vi "PROJE (1).vi"() -> ()   [LabVIEW 2017]
panel:
  in  "Kaydet":bool
  in  "Çıkış":bool
  in  "Path":path
  out "Waveform Chart":dbl(graph)
  in  "SENSOR NEVEL":dbl(slide) scale=0.0..100.0
  out "Tank":dbl(slide) scale=0.0..100.0
  out "tank  hızı":dbl
  in  "tekrar sayısı":dbl
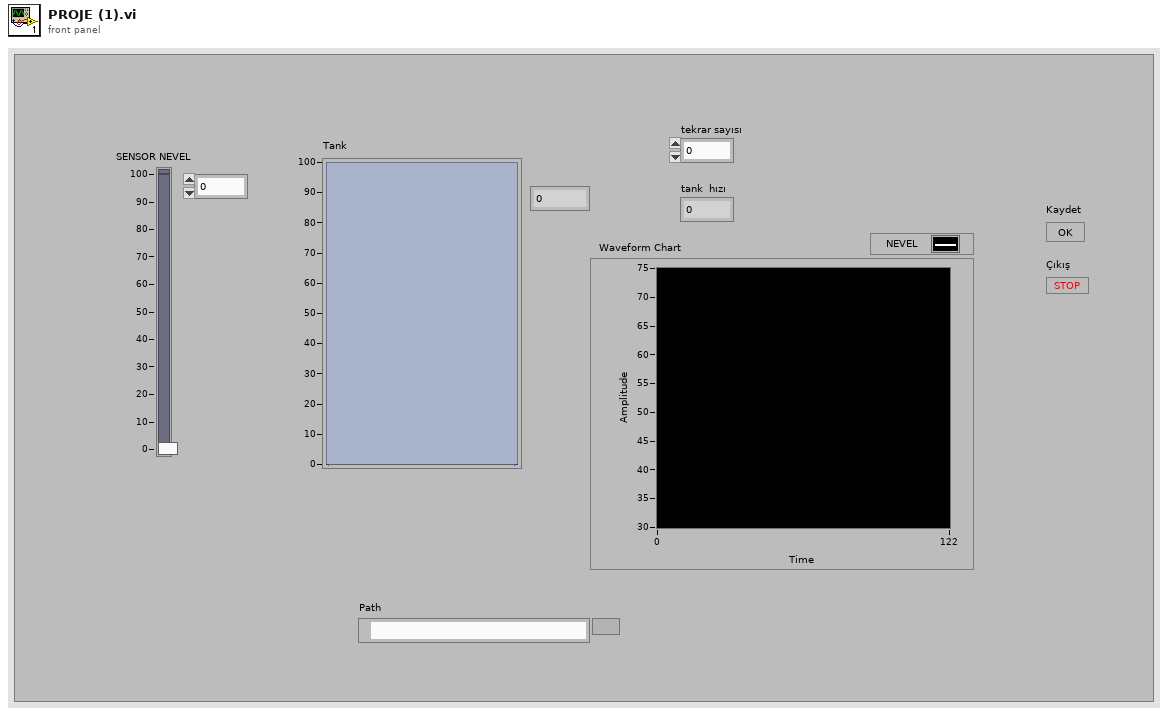
[diagram p1: front panel]
types:
  T1 = enum16{"open", "replace", "create", "open or create", "replace or create", "replace or create with confirmation"}
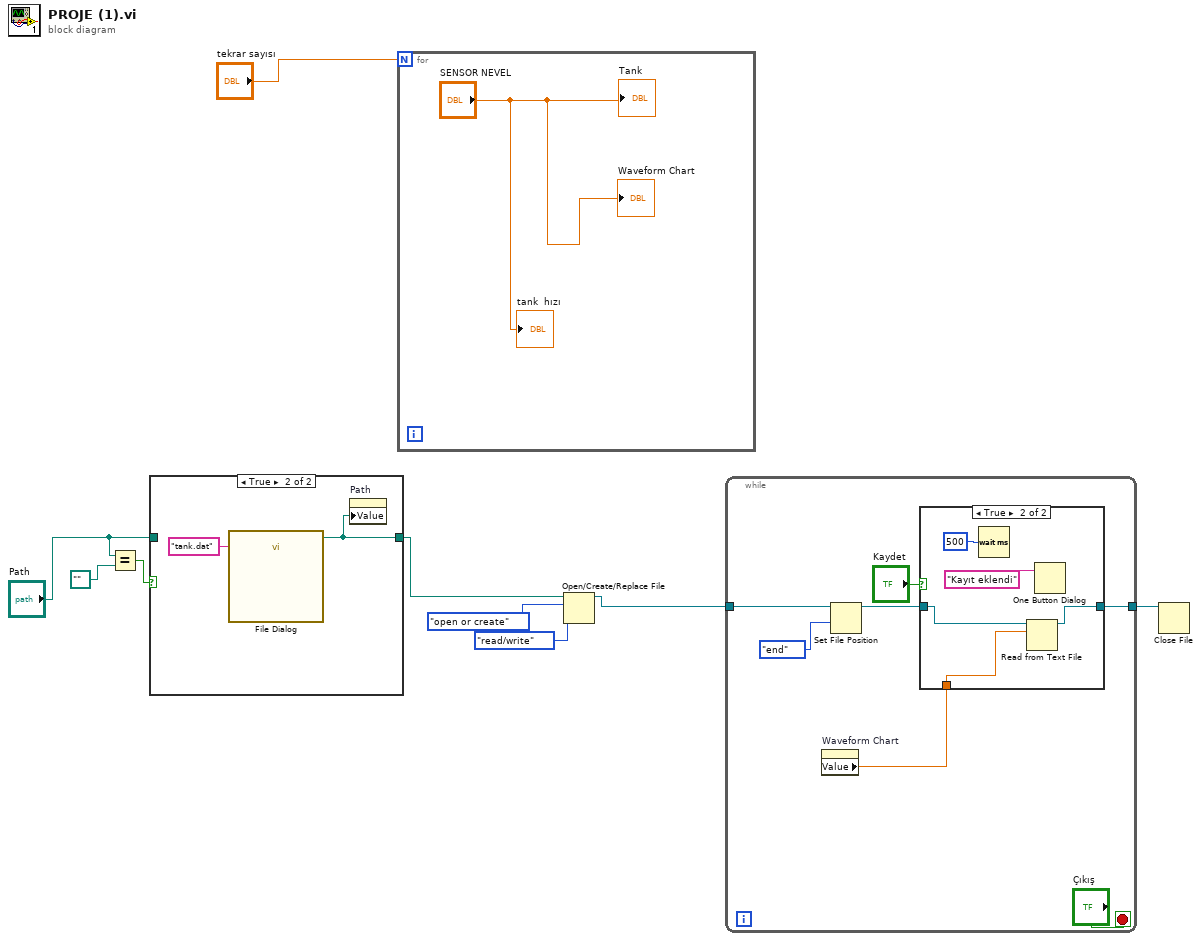
[diagram p0: block diagram]
diagram:
  n1 = Equal?(x="Path", y=path "") -> (x = y?=w8:bool)
  n2 = case shown="True" w8 {
    tunnel: [w10 w11] -> w3
    tunnel: "Path" -> [w10 _]
    frame False {
    }
    frame True {
      n3 = call "File Dialog"("default name"="tank.dat") -> ("selected path"=w11:path)  [unwired: 11 in, 3 out]
      n4 = property on="Path" class="Path"("Value"=w11) -> ()  [unwired: 2 in, 2 out]
    }
  }
  n5 = for {
    N: "tekrar sayısı" -> [_]
    "tank  hızı" <- "SENSOR NEVEL"
    "Tank" <- "SENSOR NEVEL"
    "Waveform Chart" <- "SENSOR NEVEL"
  }
  n6 = Open/Create/Replace File(file path (use dialog)=w3, operation (0:open)=T1."open or create", access (0:read/write)=enum16{"read/write", "read-only", "write-only"}."read/write") -> (refnum out=w4:refnum<file>)  [unwired: 3 in, 2 out]
  n7 = while {
    tunnel: [w16] -> w5
    tunnel: w4 -> [w15]
    stop <- "Çıkış" stop-if-true
    n8 = property on="Waveform Chart" class="WFChart (strict)"() -> ("Value"=w14:dbl)  [unwired: 2 in, 2 out]
    n9 = Set File Position(refnum=w15, from (0:start)=enum16{"start", "end", "current"}."end") -> (refnum out=w19:refnum<file>)  [unwired: 2 in, 1 out]
    n10 = case shown="True" "Kaydet" {
      tunnel: w19 -> [w21 w22]
      tunnel: [w21 w24] -> w16
      tunnel: w14 -> [_ w23]
      frame False {
      }
      frame True {
        n11 = Wait (ms)(milliseconds to wait=u32 500) -> ()  [unwired: 1 out]
        n12 = Read from Text File(file (use dialog)=w22, count=w23) -> (refnum out=w24:refnum<file>)  [unwired: 2 in, 3 out]
        n13 = One Button Dialog(message="Kayıt eklendi") -> ()  [unwired: 1 in, 1 out]
      }
    }
  }
  n14 = Close File(refnum=w5) -> ()  [unwired: 1 in, 2 out]
